vi "sm i16 read and increment.vi"(8 "error in (no error)":errorcluster, 10 "increment value":u64=8, 11 "pointer in":u64) -> (0 "error out":errorcluster, 2 "value out":i16, 3 "Shared Memory PTR out":u64)   [LabVIEW 2017, in "linuxSharedMemory.lvlib"]
uses:
  linuxSharedMemory.lvlib
  <vilib>/NI/NI Linux RT IPC/Shared Memory/Pointer Operations/Read Scalar I16.vi
  <vilib>/NI/NI Linux RT IPC/Shared Memory/Pointer Operations/In Place Read Pointer.vi
  <vilib>/NI/NI Linux RT IPC/Shared Memory/Pointer Operations/In Place Read Scalar I16.vi
  <vilib>/NI/NI Linux RT IPC/Shared Memory/Linux RT IPC.Shared Memory.lvlib
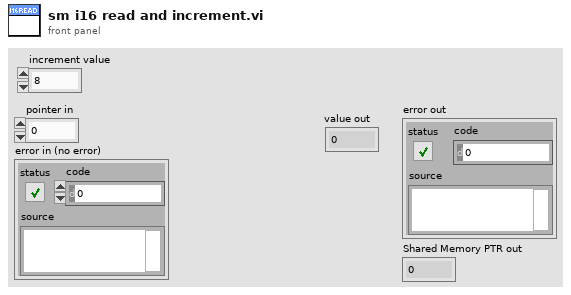
[diagram p1: front panel]
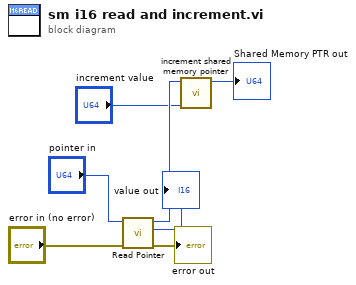
[diagram p0: block diagram]
diagram:
  n1 = call-poly <vilib>:"Read Pointer.vi"("error in (no error)"="error in (no error)", "pointer in"="pointer in") -> ("error out"=→"error out":errorcluster, "value out"=→"value out":i16, "pointer out"=w7:u64)  [unwired: 7 in]
  n2 = call "increment shared memory pointer.vi"("Increment value"="increment value", "Shared Memory PTR in"=w7) -> ("Shared Memory PTR out"=→"Shared Memory PTR out":u64)  [unwired: 9 in]
